vi "TestMemoryLeak.vi"() -> ()   [LabVIEW 2013]
panel:
  out "array type (2D Dbl)":string[](array[string])
  out "array":string[][](array[string])
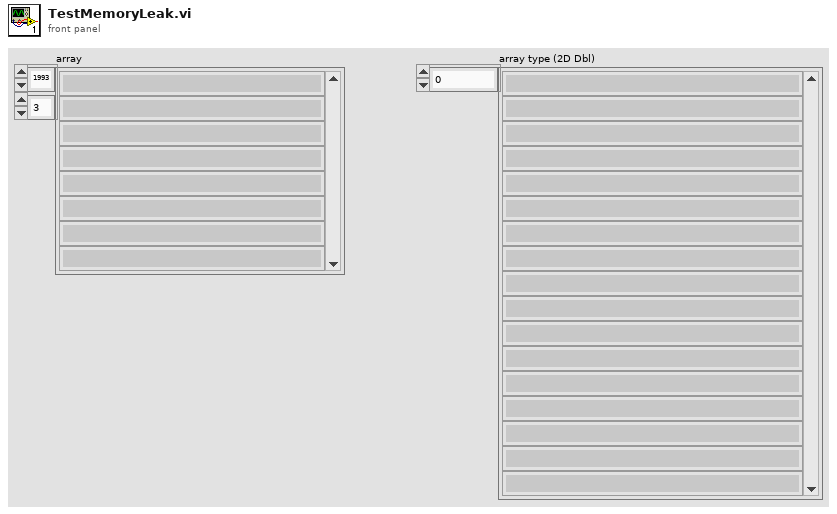
[diagram p1: front panel]
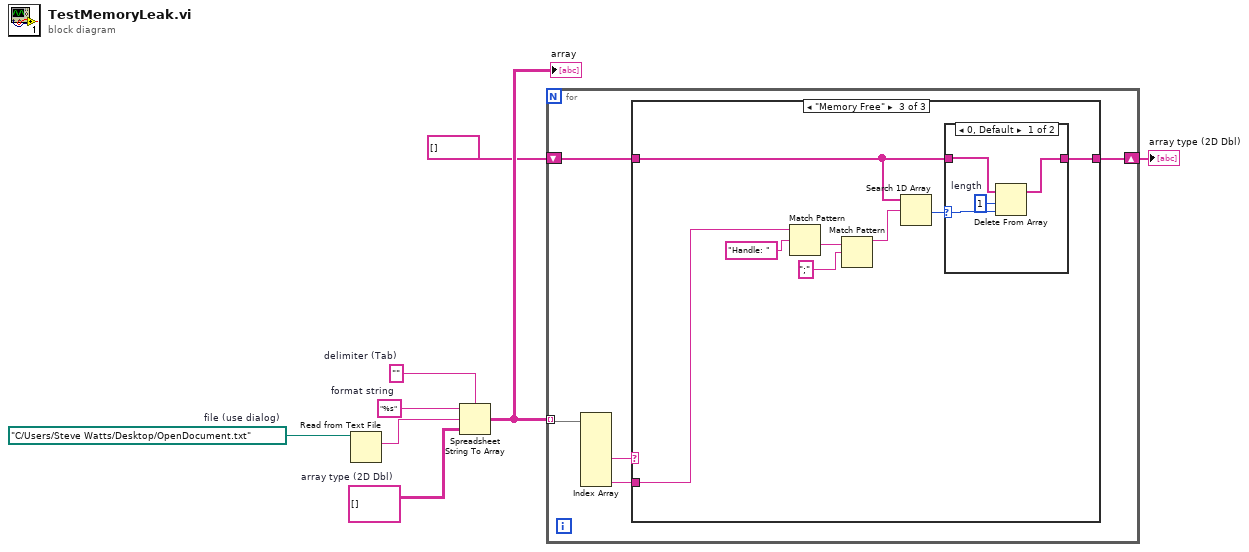
[diagram p0: block diagram]
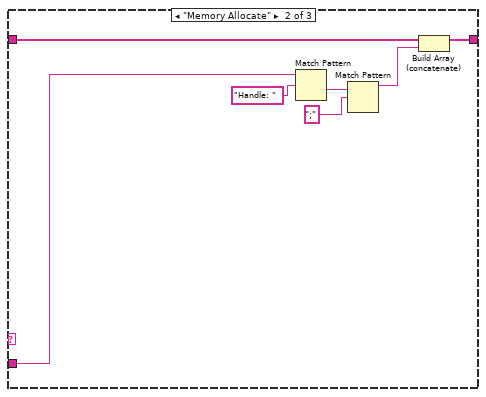
[diagram p3: hidden frame]
diagram:
  w4 = ""  # delimiter (Tab)
  w5 = "%s"  # format string
  w6 = string[][] []  # array type (2D Dbl)
  w8 = path "C:/Users/Steve Watts/Desktop/OpenDocument.txt"  # file (use dialog)
  n1 = Read from Text File(file (use dialog)=w8) -> (text=w7:string)  [unwired: 3 in, 3 out]
  n2 = Spreadsheet String To Array(delimiter (Tab)=w4, format string=w5, spreadsheet string=w7, array type (2D Dbl)=w6) -> (array=w3:string[][])
  "array" <- w3
  n3 = for {
    tunnel: w3 -> [w13] mode=indexing
    shift-right: [w9] -> w1
    shift-left: string[] [] ("array type (2D Dbl)") -> [w12]
    n4 = Index Array(array=w13) -> (element #4=w11:string, element #7=w10:string)  [unwired: 7 in, 5 out]
    n5 = case shown="\"Memory Free\"" w11 {
      tunnel: w12 -> [w14 w21 w28]
      tunnel: w10 -> [_ w16 w23]
      tunnel: [w14 w20 w27] -> w9
      frame "False", Default {
      }
      frame "Memory Allocate" {
        n6 = Match Pattern(string=w16, regular expression="Handle: ") -> (after substring=w18:string)  [unwired: 1 in, 3 out]
        n7 = Match Pattern(string=w18, regular expression=";") -> (before substring=w15:string)  [unwired: 1 in, 3 out]
        n8 = Build Array (concatenate)(w21, w15) -> (w20:string[])
      }
      frame "Memory Free" {
        n9 = Match Pattern(string=w23, regular expression="Handle: ") -> (after substring=w25:string)  [unwired: 1 in, 3 out]
        n10 = Match Pattern(string=w25, regular expression=";") -> (before substring=w22:string)  [unwired: 1 in, 3 out]
        n11 = Search 1D Array(1D array=w28, element=w22) -> (index of element=w29:i32)  [unwired: 1 in]
        n12 = case shown="0, Default" w29 {
          selector: w29 -> [w33 _]
          tunnel: w28 -> [w31 w34]
          tunnel: [w30 w34] -> w27
          frame 0, Default {
            w32 = 1  # length
            n13 = Delete From Array(array=w31, length=w32, index=w33) -> (array with subset deleted=w30:string[])  [unwired: 1 out]
          }
          frame -1 {
          }
        }
      }
    }
  }
  "array type (2D Dbl)" <- w1
